vi "Generate mounth year strings.vi"(7 "Dashes?":bool, 11 "seconds since 1904 (default 0 = now)":u32) -> (0 "mmdd":string, 3 "Month_year":string)   [LabVIEW 2015]
panel:
  out "Old result":string
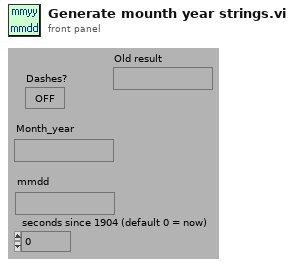
[diagram p1: front panel]
types:
  T1 = typedef "LVDateTimeRec.ctl" = cluster{"fractional second":dbl, "second":i32, "minute":i32, "hour":i32, "day of month":i32, "month":i32, "year":i32, "day of week":i32, "day of year":i32, "DST":i32}
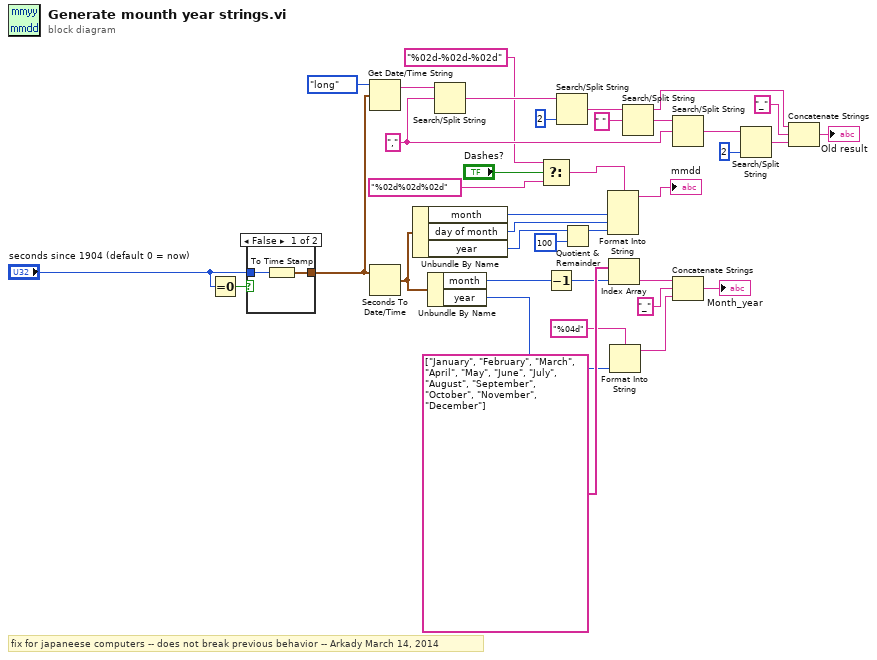
[diagram p0: block diagram]
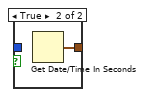
[diagram p2: hidden frame]
diagram:
  w29 = ","
  # "fix for japaneese computers -- does not break previous behavior -- Arkady March 14, 2014"
  n1 = Equal To 0?(x="seconds since 1904 (default 0 = now)") -> (x = 0?=w24:bool)
  n2 = case shown="False" w24 {
    tunnel: [w38 w40] -> w18
    tunnel: "seconds since 1904 (default 0 = now)" -> [w39 _]
    frame False {
      n3 = To Time Stamp(1:w39) -> (0:w38:timestamp)
    }
    frame True {
      n4 = Get Date/Time In Seconds() -> (seconds since 1Jan1904=w40:timestamp)
    }
  }
  n5 = Get Date/Time String(date format (0)=enum16{"short", "long", "abbreviated"}."long", seconds (now)=w18) -> (date string=w37:string)  [unwired: 2 out]
  n6 = Seconds To Date/Time(time stamp (now)=w18) -> (date time rec=w3:T1)  [unwired: 1 out]
  n7 = Unbundle By Name(w3) -> ("month"=w22:i32, "day of month"=w21:i32, "year"=w5:i32)
  n8 = Unbundle By Name(w3) -> ("month"=w7:i32, "year"=w4:i32)
  n9 = Search/Split String(string=w37, search string/char (-)=w29) -> (match + rest of string=w35:string)  [unwired: 3 out]
  n10 = Select(t="%02d-%02d-%02d", s="Dashes?", f="%02d%02d%02d") -> (s? t:f=w16:string)
  n11 = Decrement(x=w7) -> (x-1=w6:i32)
  n12 = Search/Split String(string=w35, offset (0)=2) -> (match + rest of string=w34:string)  [unwired: 3 out]
  n13 = Quotient & Remainder(x=w5, y=100) -> (x-y*floor(x/y)=w19:i32)  [unwired: 1 out]
  n14 = Format Into String(format string=w16, w22, w21, w19) -> (resulting string=→"mmdd":string)  [unwired: 2 in, 1 out]
  n15 = Index Array(array=string[] ["January", "February", "March", "April", "May", "June", "July", "August", "September", "October", "November", "December"], index=w6) -> (element=w10:string)
  n16 = Format Into String(format string="%04d", w4) -> (resulting string=w8:string)  [unwired: 2 in, 1 out]
  n17 = Search/Split String(string=w34, search string/char (-)=" ") -> (substring before match=w26:string, match + rest of string=w31:string)  [unwired: 2 out]
  n18 = Search/Split String(string=w31, search string/char (-)=w29) -> (match + rest of string=w28:string)  [unwired: 3 out]
  n19 = Concatenate Strings(w10, "_" ("substring before char"), w8) -> (→"Month_year":string)
  n20 = Search/Split String(string=w28, offset (0)=2) -> (match + rest of string=w32:string)  [unwired: 3 out]
  n21 = Concatenate Strings(w26, "_" ("substring before char"), w32) -> (→"Old result":string)
